vi "Byte Array to Single Array.vi"(11 "Byte Array":u8[](array[numeric])) -> (3 "SGL Array":sgl[](array[numeric]))   [LabVIEW 2020, in "Rover.lvlib" / "Rover.lvclass"]
uses:
  Rover.lvclass
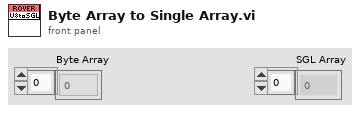
[diagram p1: front panel]
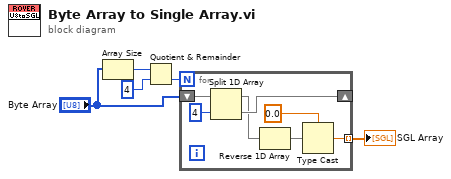
[diagram p0: block diagram]
diagram:
  n1 = Array Size(array="Byte Array") -> (size(s)=w5:i32)
  n2 = Quotient & Remainder(x=w5, y=4) -> (floor(x/y)=w3:i32)  [unwired: 1 out]
  n3 = for {
    N: w3 -> [_]
    shift-right: [w10] -> _
    shift-left: "Byte Array" -> [w12]
    tunnel: [w6] -> w1 mode=indexing
    n4 = Split 1D Array(array=w12, index=4) -> (first subarray=w9:u8[], second subarray=w10:u8[])
    n5 = Reverse 1D Array(array=w9) -> (reversed array=w8:u8[])
    n6 = Type Cast(type=sgl 0.0, x=w8) -> (*(type *) &x=w6:sgl)
  }
  "SGL Array" <- w1
